vi "Global Label.vi"() -> ()   [LabVIEW 2020]
panel:
  out "Label":dbl
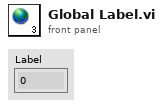
[diagram p1: front panel]
diagram:
